vi "Start Controller.vi"(8 "error in (no error)":errorcluster, 10 "Window Handle":i32, 11 "Config File Path":path=path "MeasurementConfig.ini") -> (0 "error out":errorcluster, 2 "Path to config file":path, 3 "Controller Queue":refnum<class "Message Enqueuer.lvclass">)   [LabVIEW 2015, in "Controller API.lvlib" / "Controller API.lvclass"]
doc: "This starts the controller that runs in the background to monitor running measurements and manage available resources. The path that is supplied to this method specifies the location of the configuration file. If it is not absolute, it will be appended to the disk location of this method. If the file does not exist at the specified location, it will be created using default settings."
uses:
  Controller API.lvclass
  <vilib>/ActorFramework/Message Enqueuer/Message Enqueuer.lvclass
  <userlib>/Common Components/Msmt Configuration/Controller Configuration.lvclass
  Controller API.lvclass/Controller API.ctl
  <vilib>/ActorFramework/Message Queue/Message Queue.lvclass/Message Queue.ctl
  <userlib>/Common Components/Controller/Controller.lvclass/Controller.ctl
  <userlib>/Common Components/Controller/Accessors/Write Root Path.vi
  <vilib>/ActorFramework/Actor/Actor.lvclass
  <vilib>/ActorFramework/Message Queue/Message Queue.lvclass
  <userlib>/Common Components/Controller/Controller.lvclass
  <userlib>/Configuration Dialog Actor/Configuration.lvclass
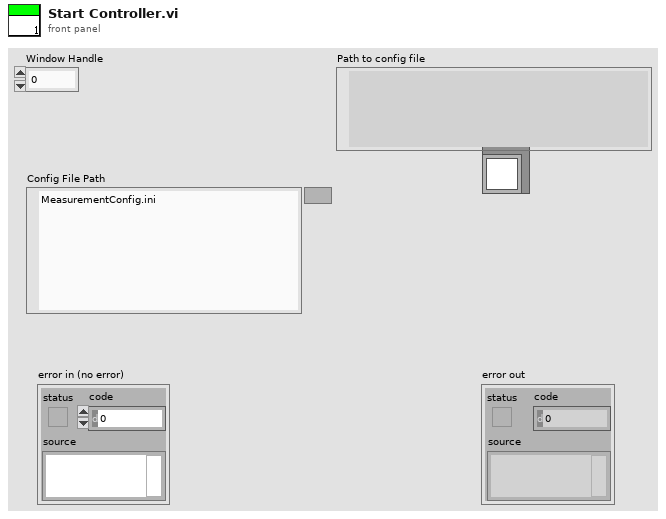
[diagram p1: front panel]
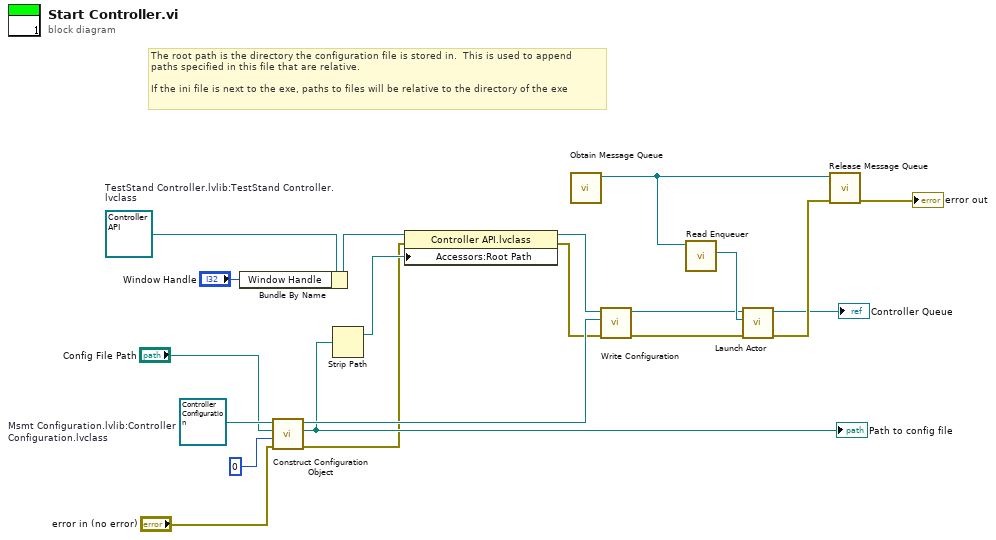
[diagram p0: block diagram]
diagram:
  w12 = refnum<class "Controller Configuration.lvclass"> refnum  # Msmt Configuration.lvlib:Controller Configuration.lvclass
  w8 = refnum<class "Controller API.lvclass"> refnum  # TestStand Controller.lvlib:TestStand Controller.lvclass
  # "The root path is the directory the configuration file is stored in.  This is used to append\npaths specified in this file that are relative.\n\nIf the ini file is next to the exe, paths to files will be relative to the directory of the exe"
  n1 = Bundle By Name(cluster=w8, "Window Handle"="Window Handle") -> (w7:refnum<class "Controller API.lvclass">)
  n2 = call <userlib>:"Construct Configuration Object.vi"("error in (no error)"="error in (no error)", "Initial Category Selection"=0, "Configuration File Path"="Config File Path", "Configuration in"=w12) -> ("error out"=w1:errorcluster, "Path to config file"=w3:path, "Configuration out"=w17:refnum<class "Controller Configuration.lvclass">)  [unwired: 4 in, 1 out]
  "Path to config file" <- w3
  n3 = Strip Path(path=w3) -> (stripped path=w9:path)  [unwired: 1 out]
  n4 = property class="Controller API.lvclass"(reference=w7, error in=w1, "Accessors:Root Path"=w9) -> (reference out=w16:refnum<class "Controller API.lvclass">, error out=w5:errorcluster)
  n5 = call <vilib>:"Obtain Message Queue.vi"() -> ("Message Queue"=w20:refnum<class "Message Queue.lvclass">)  [unwired: 10 in, 1 out]
  n6 = call <userlib>:"Write Configuration.vi"("error in (no error)"=w5, "Configuration.lvlib:Configuration.lvclass"=w17, "Controller in"=w16) -> ("error out"=w11:errorcluster, "Controller out"=w14:refnum<class "Controller API.lvclass">)  [unwired: 7 in]
  n7 = call <vilib>:"Read Enqueuer.vi"("Message Queue"=w20) -> ("Message Enqueuer"=w19:refnum<class "Message Enqueuer.lvclass">)  [unwired: 10 in]
  n8 = call <vilib>:"Launch Actor.vi"("error in (no error)"=w11, "Actor-to-Caller Enqueuer"=w19, "Actor"=w14) -> ("error out"=w18:errorcluster, "Caller-To-Actor Enqueuer"=→"Controller Queue":refnum<class "Message Enqueuer.lvclass">)  [unwired: 7 in]
  n9 = call <vilib>:"Release Message Queue.vi"("error in (no error)"=w18, "Message Queue"=w20) -> ("error out"=→"error out":errorcluster)  [unwired: 8 in, 1 out]
